vi "DriveAutoSpin.vi"(8 "Current Heading":dbl, 10 "Target Angle":dbl, 11 "Directions":T1) -> (0 "Done?":bool, 2 "Right Motor Value":dbl, 3 "Left Motor Value":dbl)   [LabVIEW 2017, in "DriveAuto.lvclass"]
uses:
  DriveAuto.lvclass
  Team-code/DriveAutoDirections.ctl
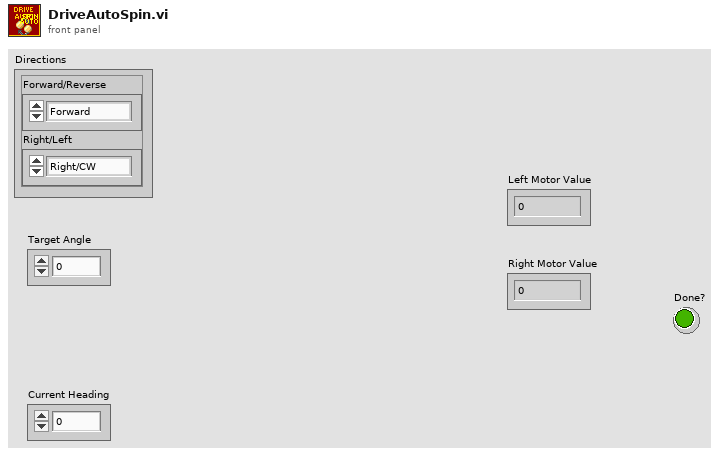
[diagram p1: front panel]
types:
  T1 = typedef "DriveAutoDirections.ctl" = cluster{"Forward/Reverse":enum16{"Forward", "Reverse"}, "Right/Left":enum16{"Right/CW", "Left/CCW"}}
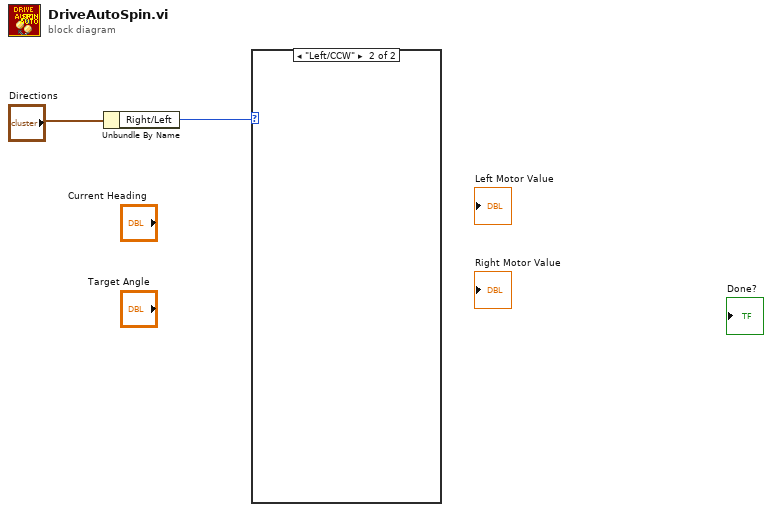
[diagram p0: block diagram]
diagram:
  n1 = Unbundle By Name("Directions") -> ("Right/Left"=w1:enum16{"Right/CW", "Left/CCW"})
  n2 = case shown="\"Left/CCW\"" w1 {
    frame "Right/CW", Default {
    }
    frame "Left/CCW" {
    }
  }
